vi "write_REC.vi"(6 "Rec":variant, 8 "error in":errorcluster, 11 "HDF5 Ref in":T1) -> (0 "error out":errorcluster, 3 "HDF5 Ref out":T1)   [LabVIEW 2015, in "oskar_tools.lvlib"]
uses:
  <vilib>/UPVI/lvhdf5/library.llb/HDF5 Ref.ctl
  <vilib>/UPVI/lvhdf5/attribute.llb/Simple H5Awrite (Variant).vi
  <vilib>/UPVI/lvhdf5/attribute.llb/LVH5A Operation.ctl
  <vilib>/UPVI/lvhdf5/attribute.llb/Simple H5Awrite.xnode
  oskar_tools.lvlib
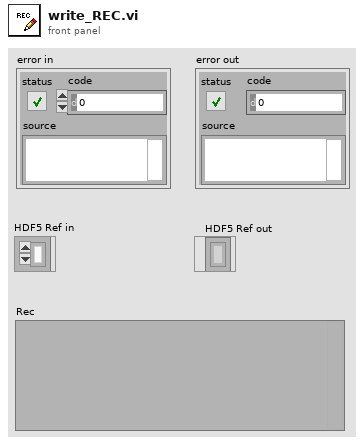
[diagram p1: front panel]
types:
  T1 = typedef "HDF5 Ref.ctl" = refnum<k1>
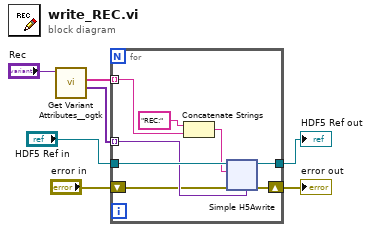
[diagram p0: block diagram]
diagram:
  n1 = call <userlib>:"Get Variant Attributes__ogtk.vi"("Variant"="Rec") -> ("value(s)"=w6:variant[], "names"=w5:string[])  [unwired: 3 in, 2 out]
  n2 = for {
    tunnel: w6 -> [w12] mode=indexing
    tunnel: w5 -> [w10] mode=indexing
    tunnel: "HDF5 Ref in" -> [w15]
    tunnel: [w14] -> w3
    shift-right: [w13] -> w2
    shift-left: "error in" -> [w11]
    n3 = Concatenate Strings("REC:" ("string"), w10) -> (w8:string)
    n4 = xnode "Simple H5Awrite"("HDF5 Ref"=w15, "Name"=w8, "error in (no error)"=w11, "Value"=w12) -> ("HDF5 Ref out"=w14:T1, "error out"=w13:errorcluster)  [unwired: 1 in]
  }
  "HDF5 Ref out" <- w3
  "error out" <- w2
